vi "RFH-average-libreVNA.vi"(5 "average filepath":path, 7 "Source Folder":path, 8 "error in (no error)":errorcluster) -> (0 "error out":errorcluster)   [LabVIEW 2020, in "RFH-Reflection_File_Handler.lvlib"]
uses:
  RFH-Reflection_File_Handler.lvlib
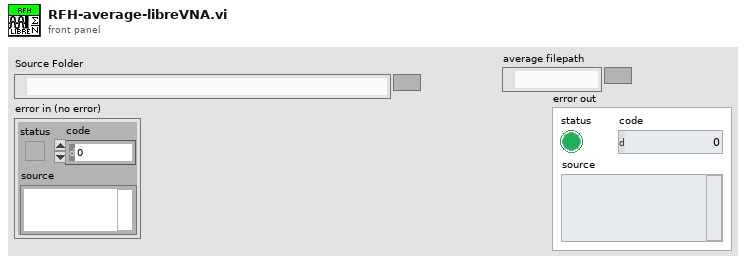
[diagram p1: front panel]
types:
  T1 = typedef "RFH-Reflection_File_Handler.lvlib/RFH-common_data_format.ctl" = cluster{"Frequency":dbl[], "Reflection'":dbl[], "Reflection''":dbl[], "Permativity'":dbl[], "Permativity''":dbl[]}
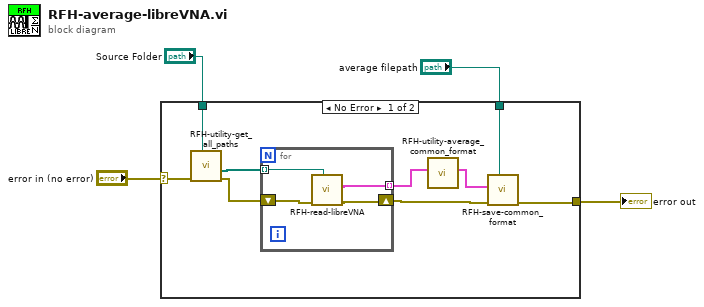
[diagram p0: block diagram]
diagram:
  n1 = case shown="No Error" "error in (no error)" {
    selector: "error in (no error)" -> [w6 w18]
    tunnel: "Source Folder" -> [w8 _]
    tunnel: "average filepath" -> [w7 _]
    tunnel: [w5 w18] -> w1
    frame No Error {
      n2 = call "RFH-utility-get_all_paths.vi"("Folder Path"=w8, "error in (no error)"=w6) -> ("error out"=w10:errorcluster, "All Files in Dir"=w13:path[])  [unwired: 6 in, 2 out]
      n3 = for {
        tunnel: w13 -> [w15] mode=indexing
        tunnel: [w14] -> w12 mode=indexing
        shift-right: [w16] -> w9
        shift-left: w10 -> [w17]
        n4 = call "RFH-read-libreVNA.vi"("file path (dialog if empty)"=w15, "error in"=w17) -> ("error out"=w16:errorcluster, "Common Format"=w14:T1)  [unwired: 8 in]
      }
      n5 = call "RFH-utility-average_common_format.vi"("common array in"=w12) -> ("Common Format"=w11:T1)  [unwired: 10 in]
      n6 = call "RFH-save-common_format.vi"("file path (use dialog)"=w7, "error in (no error)"=w9, "Common Format"=w11) -> ("error out"=w5:errorcluster)  [unwired: 8 in]
    }
    frame Error {
    }
  }
  "error out" <- w1
